vi "React Polymer.vi"(8 "Error In":errorcluster, 10 "Redux Element":string, 11 "Unreacted Polymer":string) -> (0 "Error Out":errorcluster, 2 "Size of Polymer":i32, 3 "Polymer":string)   [LabVIEW 2019]
doc: "Remove all instances of adjacent characters where their cases differ (e.g. aA bB Cc) but not where they're the same (e.g. AA bb CC).\n\nIf a redux element is provided, this VI will remove all instances of that character prior to performing the reaction."
uses:
  <vilib>/Utility/error.llb/Error Cluster From Error Code.vi
  <vilib>/ErrorRing/Error Ring.xnode
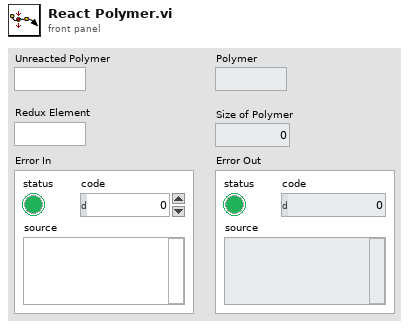
[diagram p1: front panel]
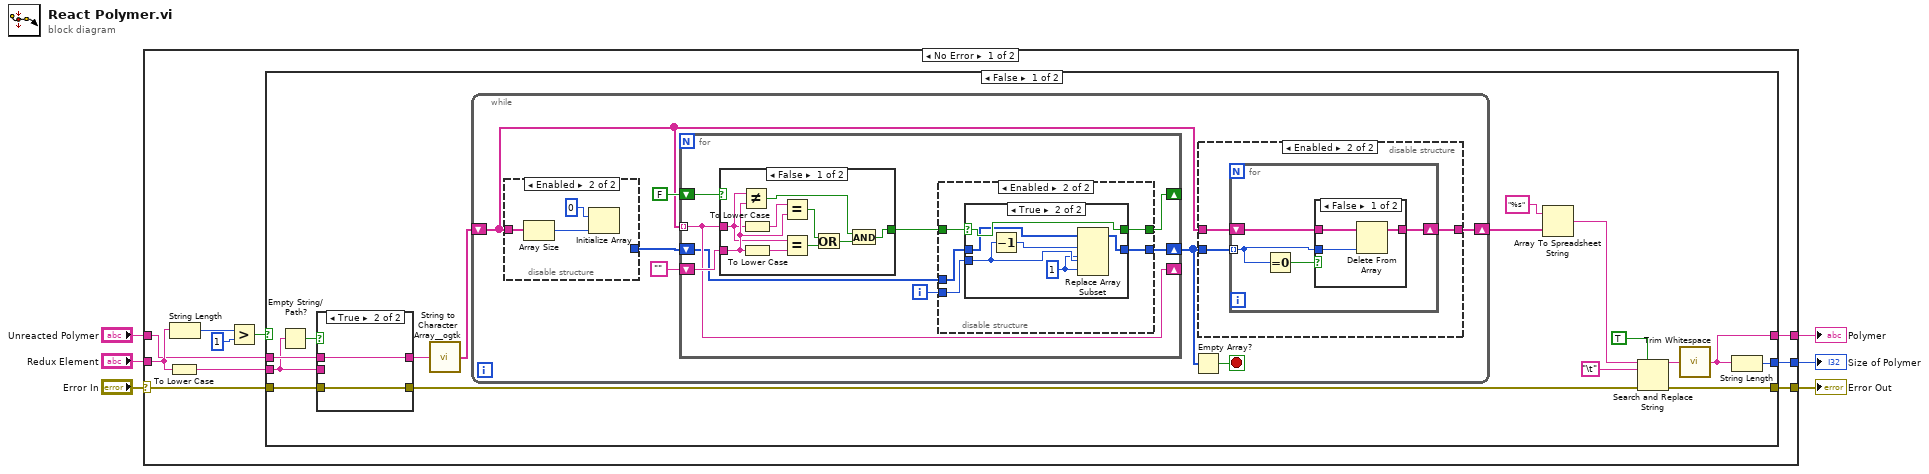
[diagram p0: block diagram]
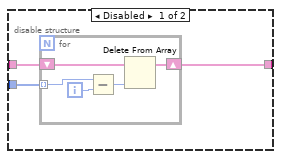
[diagram p2: hidden frame]
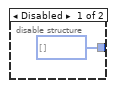
[diagram p4: hidden frame]
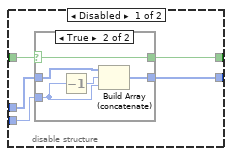
[diagram p5: hidden frame]
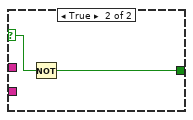
[diagram p8: hidden frame]
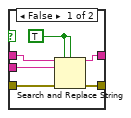
[diagram p9: hidden frame]
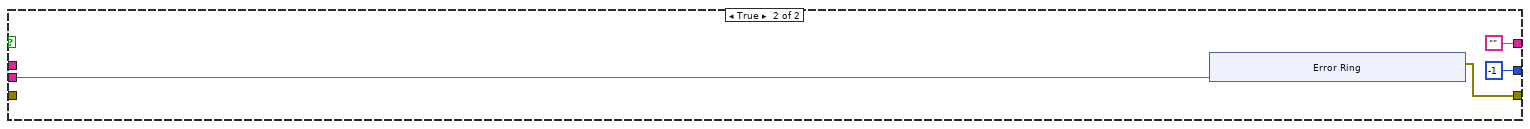
[diagram p10: hidden frame]
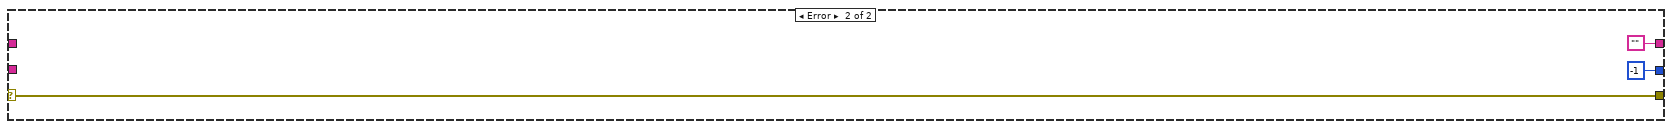
[diagram p11: hidden frame]
diagram:
  n1 = case shown="No Error" "Error In" {
    selector: "Error In" -> [w14 w126]
    tunnel: [w16 ""] -> w6
    tunnel: [w15 -1] -> w5
    tunnel: "Unreacted Polymer" -> [w7 _]
    tunnel: [w13 w126] -> w2
    tunnel: "Redux Element" -> [w11 _]
    frame No Error {
      n2 = To Lower Case(string=w11) -> (all lower case string=w12:string)
      n3 = String Length(string=w11) -> (length=w10:i32)
      n4 = Greater?(x=w10, y=1) -> (0:w8:bool)
      n5 = case shown="False" w8 {
        tunnel: [w32 ""] -> w16
        tunnel: [w30 -1] -> w15
        tunnel: w14 -> [w18 _]
        tunnel: [w24 w118] -> w13
        tunnel: w12 -> [w20 w115]
        tunnel: w7 -> [w23 _]
        frame False {
          n6 = Empty String/Path?(string/path=w20) -> (empty?=w21:bool)
          n7 = case shown="True" w21 {
            tunnel: w20 -> [w112 _]
            tunnel: w23 -> [w111 w114]
            tunnel: [w110 w114] -> w19
            tunnel: w18 -> [w109 w113]
            tunnel: [w108 w113] -> w17
            frame False {
              w107 = TRUE ("replace all? (F)")
              n8 = Search and Replace String(replace all?=w107, case sensitive?=w107, input string=w111, search string=w112, error in=w109) -> (result string=w110:string, error out=w108:errorcluster)  [unwired: 3 in, 2 out]
            }
            frame True {
            }
          }
          n9 = call <userlib>:"String to Character Array__ogtk.vi"("Input String"=w19) -> ("Character Array"=w22:string[])
          n10 = while {
            shift-right: [w34] -> w25
            shift-left: w22 -> [w33]
            stop <- w36 stop-if-true
            n11 = disable-structure shown="Enabled" {
              disable-tunnel: [i32[] [] _] -> w37
              disable-tunnel: w33 -> [_ w62]
              frame Disabled {
              }
              frame Enabled {
                n12 = Array Size(array=w62) -> (size(s)=w61:i32)
                n13 = Initialize Array(0 ("element"), w61) -> ()  [unwired: 1 out]
              }
            }
            n14 = for {
              tunnel: w33 -> [w69] mode=indexing
              shift-right: [w69] -> _
              shift-left: "" -> [w70]
              shift-right: [w66] -> _
              shift-left: FALSE -> [w68]
              shift-right: [w63] -> w35
              shift-left: w37 -> [w65]
              i -> [w64]
              n15 = case shown="False" w68 {
                selector: w68 -> [_ w106]
                tunnel: w70 -> [w104 _]
                tunnel: w69 -> [w100 _]
                tunnel: [w96 w105] -> w67
                frame False {
                  n16 = Not Equal?(x=w100, y=w104) -> (x != y?=w98:bool)
                  n17 = To Lower Case(string=w100) -> (all lower case string=w99:string)
                  n18 = To Lower Case(string=w104) -> (all lower case string=w101:string)
                  n19 = Equal?(x=w99, y=w104) -> (x = y?=w102:bool)
                  n20 = Equal?(x=w100, y=w101) -> (x = y?=w103:bool)
                  n21 = Or(x=w102, y=w103) -> (x .or. y?=w97:bool)
                  n22 = And(x=w98, y=w97) -> (x .and. y?=w96:bool)
                }
                frame True {
                  n23 = Not(x=w106) -> (.not. x?=w105:bool)
                }
              }
              n24 = disable-structure shown="Enabled" {
                disable-tunnel: w67 -> [w75 w85]
                disable-tunnel: [w74 w84] -> w66
                disable-tunnel: w65 -> [w73 w87]
                disable-tunnel: w64 -> [w72 w86]
                disable-tunnel: [w71 w83] -> w63
                frame Disabled {
                  n25 = case shown="True" w75 {
                    selector: w75 -> [w77 w82]
                    tunnel: [w77 w82] -> w74
                    tunnel: w73 -> [w76 w81]
                    tunnel: w72 -> [_ w78]
                    tunnel: [w76 w80] -> w71
                    frame False {
                    }
                    frame True {
                      n26 = Decrement(x=w78) -> (x-1=w79:i32)
                      n27 = Build Array (concatenate)(w81, w79, w78) -> (w80:i32[])
                    }
                  }
                }
                frame Enabled {
                  n28 = case shown="True" w85 {
                    selector: w85 -> [w89 w95]
                    tunnel: [w89 w95] -> w84
                    tunnel: w87 -> [w88 w94]
                    tunnel: w86 -> [_ w93]
                    tunnel: [w88 w90] -> w83
                    frame False {
                    }
                    frame True {
                      w91 = 1 ("new element/subarray")
                      n29 = Decrement(x=w93) -> (x-1=w92:i32)
                      n30 = Replace Array Subset(array=w94, new element #1=w91, index #1=w92, new element #2=w91, index #2=w93) -> (w90:i32[])
                    }
                  }
                }
              }
            }
            n31 = Empty Array?(array=w35) -> (empty?=w36:bool)
            n32 = disable-structure shown="Enabled" {
              disable-tunnel: w35 -> [w42 w49]
              disable-tunnel: [w41 w48] -> w34
              disable-tunnel: w33 -> [w40 w50]
              frame Disabled {
                n33 = for {
                  tunnel: w42 -> [w47] mode=indexing
                  shift-right: [w44] -> w41
                  shift-left: w40 -> [w45]
                  i -> [w46]
                  n34 = Subtract(x=w47, y=w46) -> (x-y=w43:i32)
                  n35 = Delete From Array(array=w45, index=w43) -> (array with subset deleted=w44:string[])  [unwired: 1 in, 1 out]
                }
              }
              frame Enabled {
                n36 = for {
                  shift-right: [w52] -> w48
                  shift-left: w50 -> [w53]
                  tunnel: w49 -> [w51] mode=indexing
                  n37 = Equal To 0?(x=w51) -> (x = 0?=w54:bool)
                  n38 = case shown="False" w54 {
                    tunnel: w53 -> [w57 w58]
                    tunnel: [w55 w58] -> w52
                    tunnel: w51 -> [w56 _]
                    frame False {
                      n39 = Delete From Array(array=w57, index=w56) -> (array with subset deleted=w55:string[])  [unwired: 1 in, 1 out]
                    }
                    frame True {
                    }
                  }
                }
              }
            }
          }
          n40 = Array To Spreadsheet String(array=w25, 3:"%s" ("format string")) -> (spreadsheet string=w28:string)  [unwired: 1 in]
          n41 = Search and Replace String(replace all?=TRUE ("replace all? (F)"), input string=w28, search string="\t", error in=w17) -> (result string=w31:string, error out=w24:errorcluster)  [unwired: 4 in, 2 out]
          n42 = call <vilib>:"Trim Whitespace.vi"("string"=w31) -> ("trimmed string"=w32:string)  [unwired: 1 in]
          n43 = String Length(string=w32) -> (length=w30:i32)
        }
        frame True {
          n44 = xnode "Error Ring"("parameter 0"=w115) -> ("error out"=w118:errorcluster)
        }
      }
    }
    frame Error {
    }
  }
  "Polymer" <- w6
  "Size of Polymer" <- w5
  "Error Out" <- w2
